vi "Write Objects.vi"(8 "error in":errorcluster, 10 "Objects":T1[](array[typedef]) {"Object ID" format="%x"}, 11 "Standard Data Model in":refnum<class "Standard Data Model.lvclass">) -> (0 "error out":errorcluster, 3 "Standard Data Model out":refnum<class "Standard Data Model.lvclass">)   [LabVIEW 2021, in "Standard Data Model.lvclass"]
doc: "Writes objects to the device model."
uses:
  Standard Data Model.lvclass
  Identification Parameters.ctl
  Standard Data Model.lvclass/Standard Data Model.ctl
  Device Data Model.lvclass
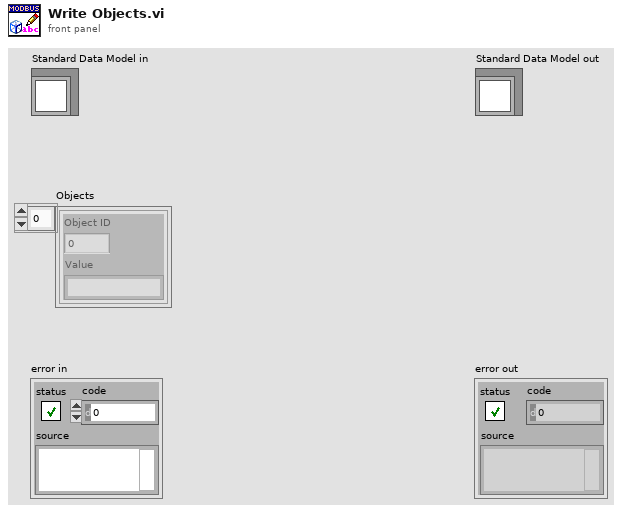
[diagram p1: front panel]
types:
  T1 = typedef "Device Data Model.lvclass/Identification Parameters.ctl" = cluster{"Object ID":u8, "Value":string}
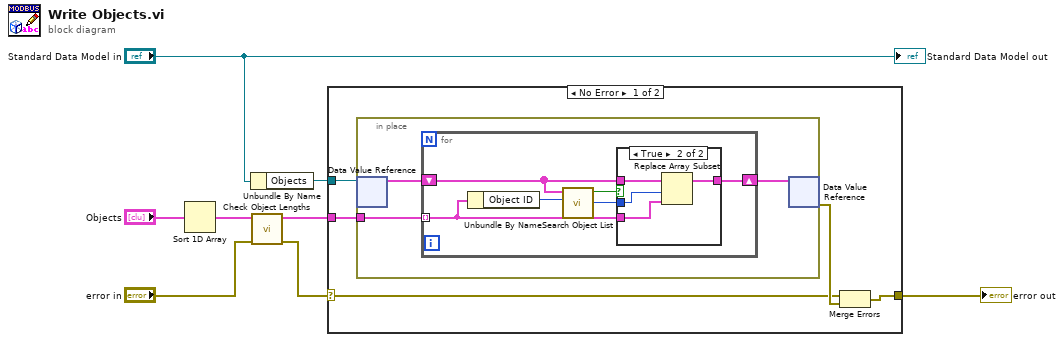
[diagram p0: block diagram]
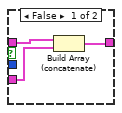
[diagram p2: hidden frame]
diagram:
  n1 = Sort 1D Array(array="Objects") -> (sorted array=w5:T1[])
  n2 = Unbundle By Name("Standard Data Model in") -> ("Objects"=w7:refnum<data-value>)
  n3 = call "Check Object Lengths.vi"("error in"="error in", "objects in"=w5) -> ("error out"=w3:errorcluster, "objects out"=w1:T1[])  [unwired: 8 in]
  n4 = case shown="No Error" w3 {
    selector: w3 -> [w9 w30]
    tunnel: [w12 w30] -> w2
    tunnel: w7 -> [w11 _]
    tunnel: w1 -> [w10 _]
    frame No Error {
      n5 = in-place {
        in-place-border: w10 -> [w14]
        n6 = in-place-dvr #1(w11) -> (w16:T1[])  [unwired: 1 out]
        n7 = for {
          shift-right: [w18] -> w15
          shift-left: w16 -> [w19]
          tunnel: w14 -> [w17] mode=indexing
          n8 = Unbundle By Name(w17) -> ("Object ID"=w22:u8)
          n9 = call "Search Object List.vi"("Object ID"=w22, "Objects"=w19) -> ("Found?"=w21:bool, "Index"=w20:i32)  [unwired: 7 in, 1 out]
          n10 = case shown="True" w21 {
            tunnel: w17 -> [w23 w26]
            tunnel: w20 -> [_ w27]
            tunnel: w19 -> [w25 w29]
            tunnel: [w24 w28] -> w18
            frame False {
              n11 = Build Array (concatenate)(w25, w23) -> (w24:T1[])
            }
            frame True {
              n12 = Replace Array Subset(array=w29, new element=w26, index=w27) -> (w28:T1[])
            }
          }
        }
        n13 = in-place-dvr #1(w15) -> (w13:errorcluster)  [unwired: 1 out]
      }
      n14 = Merge Errors(w9, w13) -> (w12:errorcluster)
    }
    frame Error {
    }
  }
  "error out" <- w2
  "Standard Data Model out" <- "Standard Data Model in"
